vi "Write ListItemObjects.vi"(8 "error in (no error)":errorcluster, 10 "AnalysisObjects":refnum<class "AnalysisListItems.lvclass">[](array[class]), 11 "AnalysisList in":refnum<class "AnalysisList.lvclass">) -> (0 "error out":errorcluster, 3 "AnalysisList out":refnum<class "AnalysisList.lvclass">)   [LabVIEW 2017, in "AnalysisList.lvclass"]
uses:
  AnalysisList.lvclass
  AnalysisListItems/AnalysisListItems.lvclass
  AnalysisList.lvclass/AnalysisList.ctl
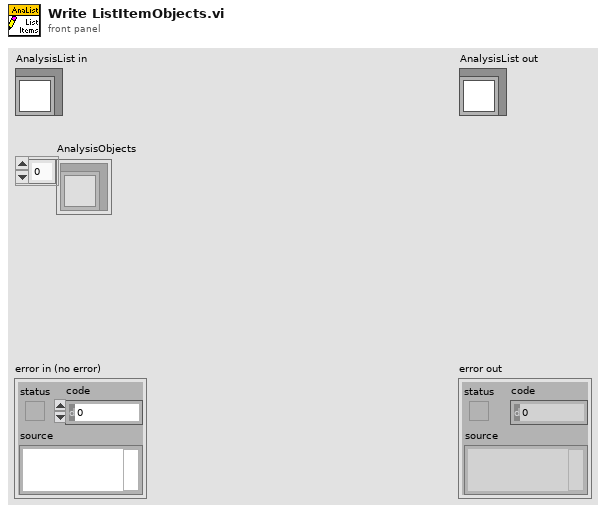
[diagram p1: front panel]
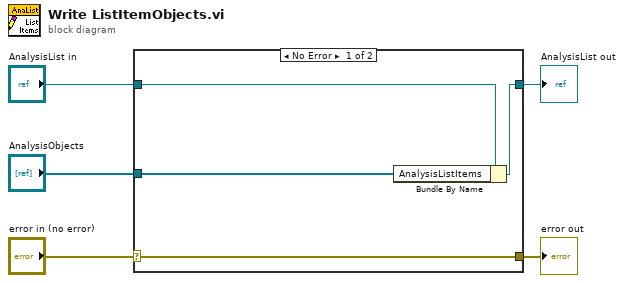
[diagram p0: block diagram]
diagram:
  n1 = case shown="No Error" "error in (no error)" {
    selector: "error in (no error)" -> [w9 w10]
    tunnel: [w9 w10] -> w4
    tunnel: [w7 w11] -> w2
    tunnel: "AnalysisList in" -> [w8 w11]
    tunnel: "AnalysisObjects" -> [w6 _]
    frame No Error {
      n2 = Bundle By Name(cluster=w8, "AnalysisListItems"=w6) -> (w7:refnum<class "AnalysisList.lvclass">)
    }
    frame Error {
    }
  }
  "error out" <- w4
  "AnalysisList out" <- w2
